vi "Memory.Pointer.Swap.vi"   [LabVIEW 2016, in "Memory Manager.lvlib" / "Memory.Pointer.lvclass"]
uses:
  Memory.Pointer.lvclass
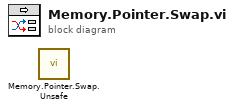
[diagram p0: block diagram]
diagram:
  n1 = call "Memory.Pointer.Swap.Unsafe.vi"() -> ()  [unwired: 9 in, 3 out]
